vi "Destroy Windows.vi"(8 "error in (no error)":errorcluster, 11 "[MDI] Parent in":refnum<class "[MDI] Parent.lvclass">) -> (0 "error out":errorcluster, 3 "[MDI] Parent out":refnum<class "[MDI] Parent.lvclass">)   [LabVIEW 2020, in "[MDI] Parent.lvlib" / "[MDI] Parent.lvclass"]
uses:
  [MDI] Parent.lvclass
  [MDI] Parent.lvclass/[MDI] Parent.ctl
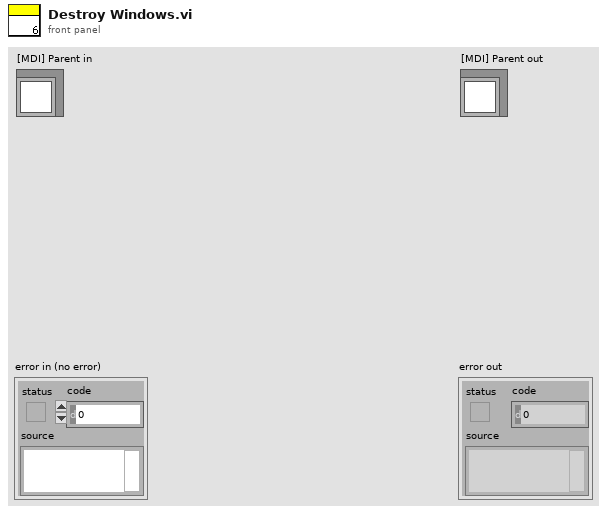
[diagram p1: front panel]
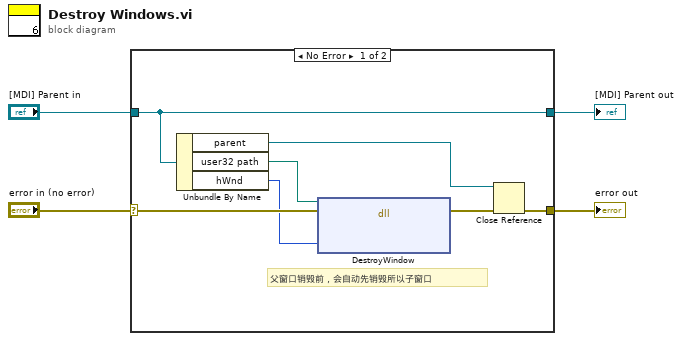
[diagram p0: block diagram]
diagram:
  n1 = case shown="No Error" "error in (no error)" {
    selector: "error in (no error)" -> [w11 w13]
    tunnel: [w6 w13] -> w3
    tunnel: [w10 w12] -> w1
    tunnel: "[MDI] Parent in" -> [w10 w12]
    frame No Error {
      # "父窗口销毁前，会自动先销毁所以子窗口"
      n2 = Unbundle By Name(w10) -> ("parent"=w7:refnum<k24>, "user32 path"=w5:path, "hWnd"=w9:u32)
      n3 = dll-call lib="user32.dll" fn="DestroyWindow"(path in=w5, error in=w11, "hWnd"=w9) -> (error out=w8:errorcluster)  [unwired: 3 in, 1 out]
      n4 = Close Reference(reference=w7, error in (no error)=w8) -> (error out=w6:errorcluster)
    }
    frame Error {
    }
  }
  "error out" <- w3
  "[MDI] Parent out" <- w1
